vi "Room API Test.vi"() -> ()   [LabVIEW 2015]
uses:
  NurseStation/TypeDef/SelectedRoom.ctl
  LVClasses/Flags/ColorFlags.ctl
  LVClasses/Request/PersonnelType.ctl
  LVClasses/Request/RequestType.ctl
  LVRestAPI/TypeDef/FGVAction.ctl
  LVRestAPI/RoomRestApi.lvlib
  LVClasses/Room/Room.lvclass
  LVClasses/Request/Request.lvclass
  LVClasses/Flags/Flags.lvclass
panel:
  in  "Request Type":T1
  in  "Personnel Type":T2 items=["Nurse", "Doctor", "Cleanning", "Admin"]
  in  "PUID":string
  in  "Flags":bool[](array[boolean])
  out "Response":string
  out "Error Out":errorcluster
  out "Selected Room":T3={"Room Number"=0, "RoomNumFlags"={"Flag State"=[1, 3, 5, 7]}, "BedVacant"=FALSE, "InRoomPersonnel"=[], "RoomRequests"=[]}
  in  "Refresh Button":bool
  in  "Room":i32
  in  "Remove Request":bool
  in  "Add Request":bool
  in  "stop":bool
  in  "URL":string="http://127.0.0.1:8001/RivERWebService/"
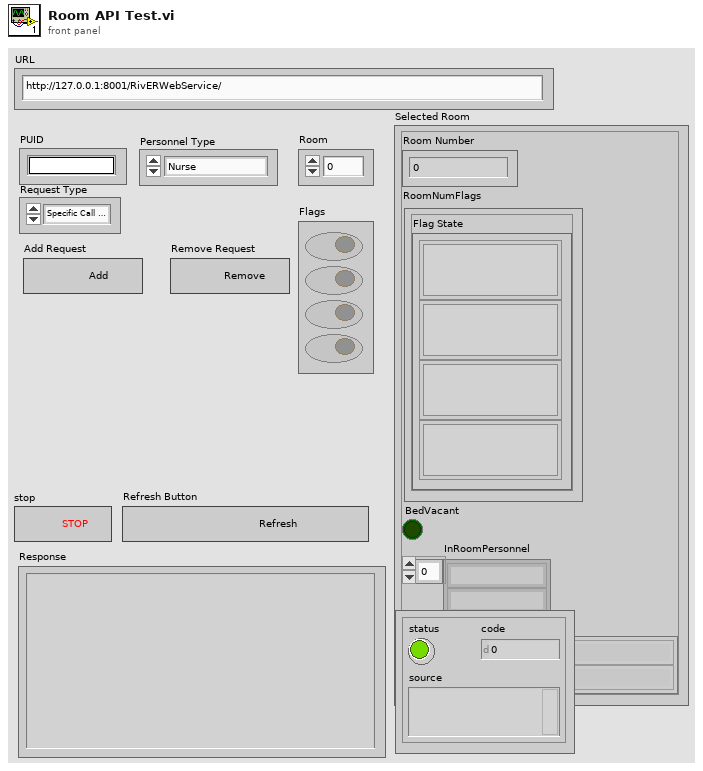
[diagram p1: front panel]
types:
  T1 = typedef "Request.lvclass/RequestType.ctl" = enum16{"Specific Call To Room", "General Call To Room"}
  T2 = typedef "Request.lvclass/PersonnelType.ctl" = u16
  T3 = typedef "Room.lvclass/SelectedRoom.ctl" = cluster{"Room Number":u8, "RoomNumFlags":T4, "BedVacant":bool, "InRoomPersonnel":string[], "RoomRequests":string[]}
  T4 = typedef "Flags.lvclass/ColorFlags.ctl" = cluster{"Flag State":u8[]}
  T5 = typedef "RoomRestApi.lvlib/FGVAction.ctl" = enum16{"Get", "Set"}
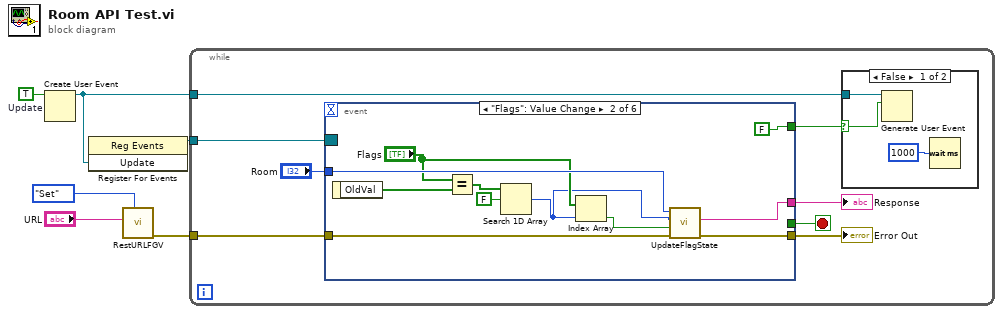
[diagram p0: block diagram]
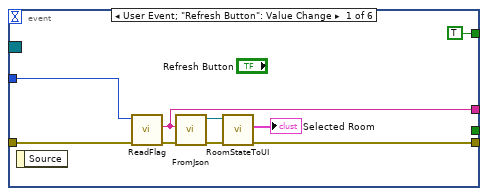
[diagram p3: hidden frame]
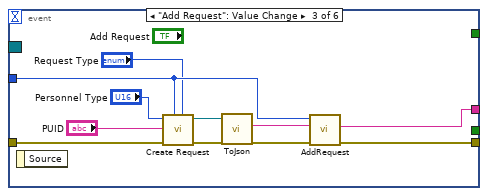
[diagram p4: hidden frame]
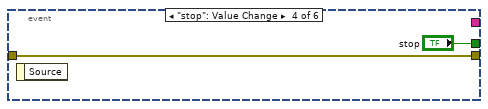
[diagram p5: hidden frame]
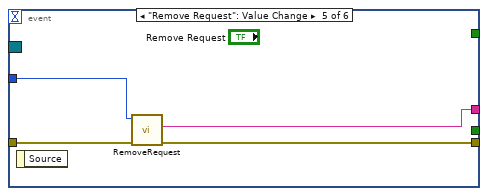
[diagram p6: hidden frame]
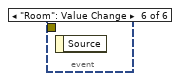
[diagram p7: hidden frame]
diagram:
  w3 = TRUE  # Update
  n1 = Create User Event(user event datatype=w3) -> (user event=w2:refnum<user-event>)  [unwired: 1 in, 1 out]
  n2 = register-events(w2) -> (reference out=w1:refnum<event-registration>)  [unwired: 2 in, 1 out]
  n3 = call "RestURLFGV.vi"("Action"=FGVAction."Set", "URL"="URL") -> ("error out"=w4:errorcluster)  [unwired: 8 in, 1 out]
  n4 = while {
    tunnel: w4 -> [w13]
    tunnel: w2 -> [w8]
    tunnel: w1 -> [w7]
    stop <- w10 stop-if-true
    n5 = event shown="[1] \"Flags\": Value Change" {
      selector: w7 -> [_ _ _ _ _ _]
      dyn-events: _ -> [_ _ _ _ _ _]
      timeout: _ -> [_ _ _ _ _ _]
      tunnel: "Room" -> [w26 w37 w45 _ w54 _]
      tunnel: w13 -> [w23 w34 w46 w49 w53 _]
      tunnel: [w20 w35 w47 w49 w52 _] -> w12
      tunnel: [w19 w36 w48 _ w51 _] -> w11
      tunnel: [_ _ _ "stop" _ _] -> w10
      tunnel: [TRUE FALSE _ _ _ _] -> w9
      event User Event; "Refresh Button": Value Change {
        n6 = event-data() -> ()  [unwired: 1 in, 1 out]
        n7 = call "ReadFlag.vi"("error in (no error)"=w23, "Room Number"=w26) -> ("error out"=w22:errorcluster, "Flags JSON"=w19:string)  [unwired: 8 in]
        n8 = call "FromJson.vi"("error in (no error)"=w22, "String"=w19) -> ("error out"=w21:errorcluster, "Room out"=w25:refnum<class "Room.lvclass">)  [unwired: 8 in]
        n9 = call "RoomStateToUI.vi"("error in"=w21, "Room In"=w25) -> ("error out"=w20:errorcluster, "Selected Room"=→"Selected Room":T3)  [unwired: 7 in, 1 out]
      }
      event "Flags": Value Change {
        n10 = event-data() -> ("OldVal"=w32:bool[])  [unwired: 1 in]
        n11 = Equal?(x="Flags", y=w32) -> (x = y?=w31:bool[])
        n12 = Search 1D Array(1D array=w31, element=FALSE) -> (index of element=w27:i32)  [unwired: 1 in]
        n13 = Index Array(array="Flags", index=w27) -> (element=w28:bool)
        n14 = call "UpdateFlagState.vi"("error in (no error)"=w34, "State"=w28, "Index"=w27, "Room Number"=w37) -> ("error out"=w35:errorcluster, "Response"=w36:string)  [unwired: 6 in]
      }
      event "Add Request": Value Change {
        n15 = event-data() -> ()  [unwired: 1 in, 1 out]
        n16 = call "Create Request.vi"("Request Type"="Request Type", "Room Number"=w45, "error in (no error)"=w46, "Name"="PUID", "Personnel Type"="Personnel Type") -> ("error out"=w44:errorcluster, "Request out"=w42:refnum<class "Request.lvclass">)  [unwired: 4 in, 1 out]
        n17 = call "ToJson.vi"("error in (no error)"=w44, "Request"=w42) -> ("error out"=w43:errorcluster, "Request"=w41:string)  [unwired: 8 in]
        n18 = call "AddRequest.vi"("error in (no error)"=w43, "Request"=w41, "Room Number"=w45) -> ("error out"=w47:errorcluster, "Response"=w48:string)  [unwired: 7 in]
      }
      event "stop": Value Change {
        n19 = event-data() -> ()  [unwired: 1 in, 1 out]
      }
      event "Remove Request": Value Change {
        n20 = event-data() -> ()  [unwired: 1 in, 1 out]
        n21 = call "RemoveRequest.vi"("error in (no error)"=w53, "Room Number"=w54) -> ("error out"=w52:errorcluster, "Response"=w51:string)  [unwired: 8 in]
      }
      event "Room": Value Change {
        n22 = event-data() -> ()  [unwired: 1 in, 1 out]
      }
    }
    "Response" <- w11
    "Error Out" <- w12
    n23 = case shown="False" w9 {
      selector: w9 -> [w15 _]
      tunnel: w8 -> [w16 _]
      frame False {
        n24 = Generate User Event(user event=w16, event data cluster=w15) -> ()  [unwired: 2 in, 2 out]
        n25 = Wait (ms)(milliseconds to wait=u32 1000) -> ()  [unwired: 1 out]
      }
      frame True {
      }
    }
  }
